vi "Kinesis - KPZ101 - Waveform LUT.vi"() -> ()   [LabVIEW 2012]
uses:
  U:/Kinesis LabVIEW Website Examples/Thorlabs.MotionControl.Controls.dll
  Thorlabs.MotionControl.Controls.dll
  U:/Kinesis LabVIEW Website Examples/Thorlabs.MotionControl.GenericPiezoCLI.dll
  Thorlabs.MotionControl.GenericPiezoCLI.dll
  <vilib>/measure/NI_MABase.lvlib
  U:/Kinesis LabVIEW Website Examples/Thorlabs.MotionControl.KCube.PiezoCLI.dll
  Thorlabs.MotionControl.KCube.PiezoCLI.dll
panel:
  in  "?":bool
  in  "?":bool
  in  "Milliseconds to Stop":u32=10000
  out "Sine Wave Array":dbl[](array[numeric])
  in  "Peak Voltage":dbl=5.0
  in  "SerialNumber":string
  in  "NumberOfCycles":u32
  in  "Mode":i16(ring)=1 items=["Continuous"=1, "Fixed"=2, "OutputTrigEnable"=4, "InputTrigEnable"=8, "OutputTrigSenseHigh"=16, "InputTrigSenseHigh"=32, "OutputGated"=64, "OutputTrigRepeat"=128]
  in  "LUTValDelay":u32=10
  in  "PostCycleDelay":u32=5
  in  "PreCycleDelay":u32=5
  in  "KCubePiezoControl":refnum<k24>(container)
  # "Notes:"
  # "- Ensure that the appropriate .DLLs are copied into your Project Folder. Check that the correct bit type are used depending on your version of LabVIEW\ni.e. 32-bit or 64-bit.\n\n\n\n\n\n\n\n\n\n\n\n\n\n\n- Open the example VI through the LabVIEW Project Explorer to correctly load the User Interface from Thorlabs.MotionControl.Controls.dll."
  # "Thorlabs Hardware: KPZ101 - K-Cube Piezo Controller\nhttps://www.thorlabs.com/newgrouppage9.cfm?objectgroup_id=2421&pn=KPZ101\n\nDescription: This VI will enable you to make use of the LUTWave Functionality available to Piezo actuated device. \nTaking advantage of the built-in Sine Waveform.vi of LabVIEW, we produce an array of sine wave component values, \nscaled by the Peak Voltage parameter below to produce our waveform. The sine wave period is represented by 50 indexed values in the array.\nUsers are then prompted to select parameters of the LUTWaveParams() struct below the UI before initiating the waveform by clicking 'GO'.\nThe below settings will output the waveform continuously until a 10 second timer has elapsed.\n\nInstructions: \n1) Connect your KPZ101 device to your PC & ensure it is powered on & the Output Enabled. \nFor full device setup, the device product manual can be found on our website here. - https://www.thorlabs.com/thorproduct.cfm?partnumber=KPZ101 \n2) Enter the device serial number below.\n3) Click 'Run' in the LabVIEW Toolbar.\n4) Assign a timer for 'Milliseconds to Stop' as a timeout for when the Waveform should stop.\n5) Assign Parameters to the Waveform & then Click 'GO' - this will print the sine wave array to the front panel & then start the waveform output.\n6) Click 'STOP' to end the program."
  # "Example Image of .NET Controller - VI opened via Project Explorer/ not opened via Project Explorer"
  # "VI Not Opened via Project Explorer"
  # "VI Opened via Project Explorer"
  # "Time before next cycle starts"
  # "Number of times to repeat cycles"
  # "- To explore the range of methods available, please visit the .NET API, included with your Kinesis software.\n\n- For tips on building your own VIs with Thorlabs Motion Control Hardware, please see our LabVIEW Guide here.\nhttps://www.thorlabs.com/newgrouppage9.cfm?objectgroup_id=10285"
  # "Time after cycle finishes"
  # "Time between output updates"
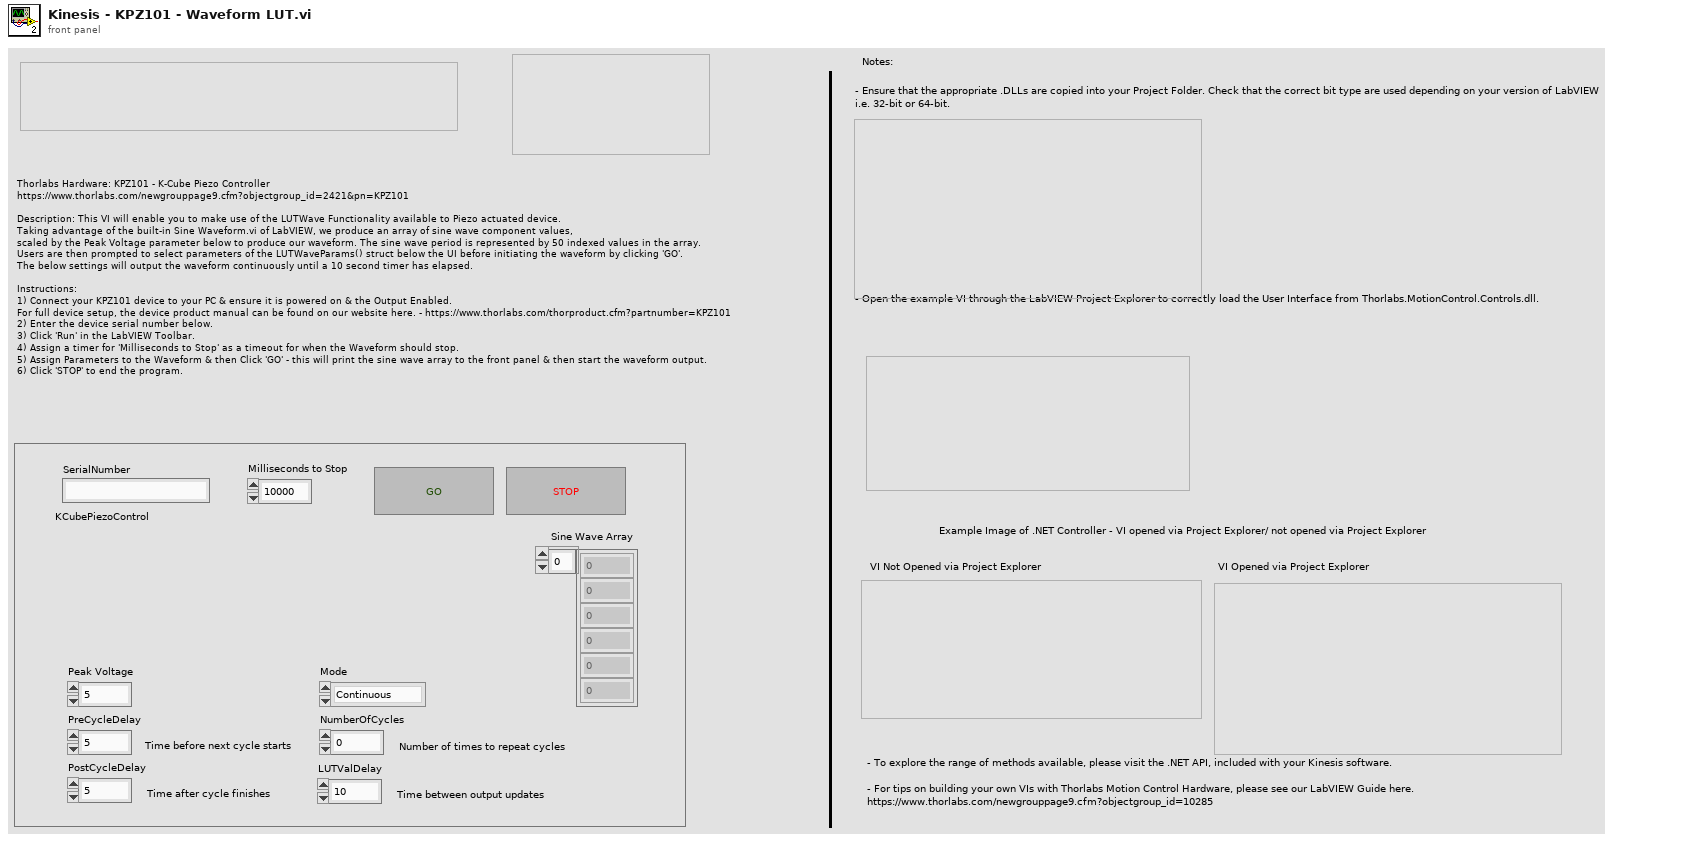
[diagram p1: front panel]
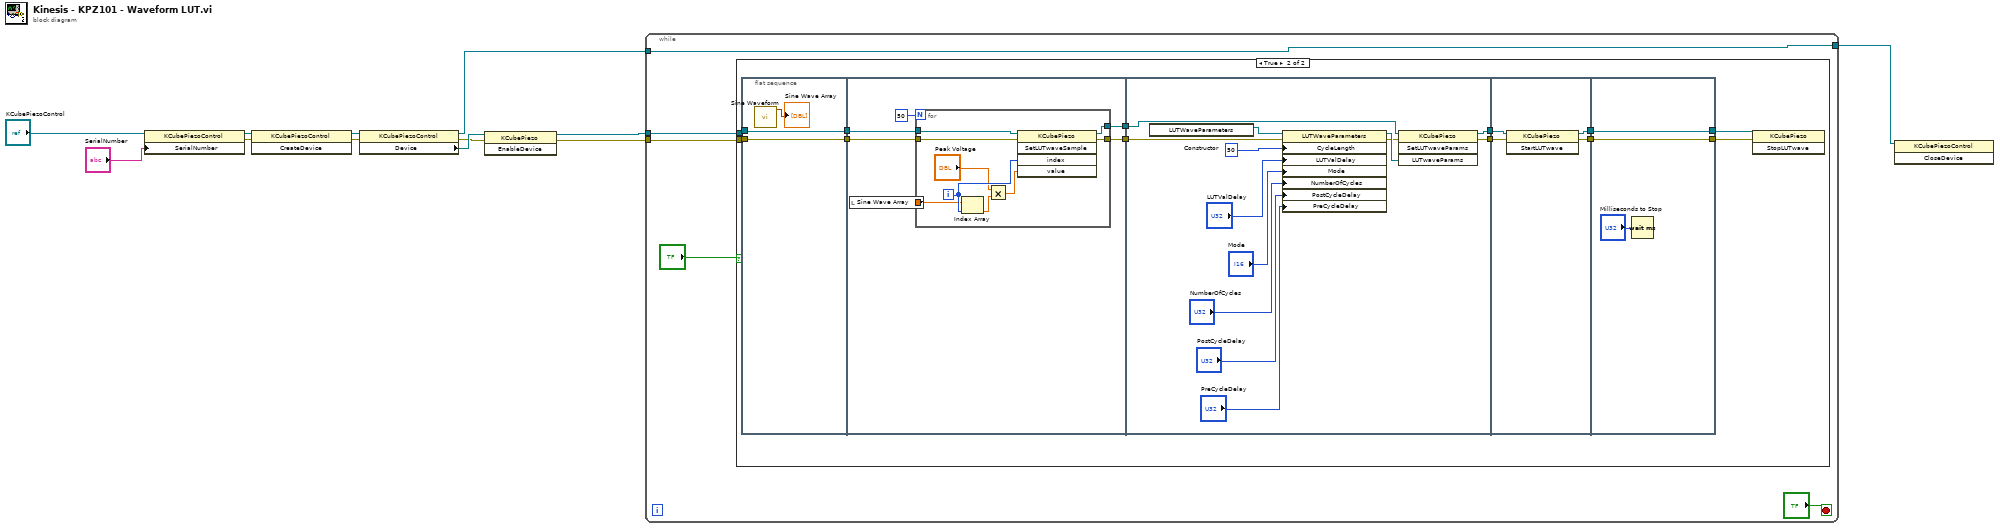
[diagram p0: block diagram]
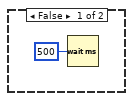
[diagram p2: hidden frame]
diagram:
  n1 = property class="KCubePiezoControl"(reference="KCubePiezoControl", "SerialNumber"="SerialNumber") -> (reference out=w11:refnum<k24>, error out=w7:errorcluster)  [unwired: 1 in]
  n2 = invoke class="KCubePiezoControl" method="CreateDevice"(reference=w11, error in=w7) -> (reference out=w10:refnum<k24>, error out=w6:errorcluster)  [unwired: 1 in, 1 out]
  n3 = property class="KCubePiezoControl"(reference=w10, error in=w6) -> (reference out=w4:refnum<k24>, error out=w5:errorcluster, "Device"=w9:refnum<k24>)
  n4 = invoke class="KCubePiezo" method="EnableDevice"(reference=w9, error in=w5) -> (reference out=w2:refnum<k24>, error out=w1:errorcluster)  [unwired: 1 in, 1 out]
  n5 = while {
    tunnel: w4 -> [w16]
    tunnel: [w16] -> w3
    tunnel: w2 -> [w15]
    tunnel: w1 -> [w14]
    stop <- "?" stop-if-true
    n6 = case shown="True" "?" {
      tunnel: w15 -> [_ w20]
      tunnel: w14 -> [_ w19]
      frame False {
        n7 = Wait (ms)(milliseconds to wait=u32 500) -> ()  [unwired: 1 out]
      }
      frame True {
        n8 = flat-sequence {
          tunnel: w20 -> [w33]
          tunnel: [w33] -> w30
          tunnel: [w31] -> w29
          tunnel: w19 -> [w31]
          tunnel: [w36] -> w28
          tunnel: w30 -> [w37]
          tunnel: w29 -> [w35]
          tunnel: [w34] -> w27
          tunnel: w28 -> [w55]
          tunnel: [w61] -> w26
          tunnel: w27 -> [w52]
          tunnel: [w50] -> w25
          tunnel: w26 -> [w65]
          tunnel: w25 -> [w63]
          tunnel: [w64] -> w24
          tunnel: [w62] -> w23
          tunnel: [w67] -> w21
          tunnel: [w68] -> w22
          tunnel: w24 -> [w68]
          tunnel: w23 -> [w67]
          frame #0 {
            n9 = call <vilib>:"Sine Waveform.vi"() -> ("signal out"=→"Sine Wave Array":waveform(dbl))  [unwired: 10 in, 1 out]
          }
          frame #1 {
            n10 = local read "Sine Wave Array"() -> (w38:dbl[])
            n11 = for {
              N: 50 -> [_]
              tunnel: w37 -> [w45]
              tunnel: [w44] -> w36
              tunnel: w35 -> [w42]
              tunnel: [w41] -> w34
              tunnel: w38 -> [w40]
              i -> [w48]
              n12 = Index Array(array=w40, index=w48) -> (element=w47:dbl)
              n13 = Multiply(x="Peak Voltage", y=w47) -> (x*y=w43:dbl)
              n14 = invoke class="KCubePiezo" method="SetLUTwaveSample"(reference=w45, error in=w42, "index"=w48, "value"=w43) -> (reference out=w44:refnum<k24>, error out=w41:errorcluster)  [unwired: 1 in, 3 out]
            }
          }
          frame #2 {
            n15 = constructor class="LUTWaveParameters"() -> (reference out=w53:refnum<k24>)  [unwired: 3 in, 2 out]
            n16 = property class="LUTWaveParameters"(reference=w53, error in=w52, "CycleLength"=i16 50, "LUTValDelay"="LUTValDelay", "Mode"="Mode", "NumberOfCycles"="NumberOfCycles", "PostCycleDelay"="PostCycleDelay", "PreCycleDelay"="PreCycleDelay") -> (reference out=w54:refnum<k24>, error out=w51:errorcluster)
            n17 = invoke class="KCubePiezo" method="SetLUTwaveParams"(reference=w55, error in=w51, "LUTwaveParams"=w54) -> (reference out=w61:refnum<k24>, error out=w50:errorcluster)  [unwired: 1 in, 2 out]
          }
          frame #3 {
            n18 = invoke class="KCubePiezo" method="StartLUTwave"(reference=w65, error in=w63) -> (reference out=w64:refnum<k24>, error out=w62:errorcluster)  [unwired: 1 in, 1 out]
          }
          frame #4 {
            n19 = Wait (ms)(milliseconds to wait="Milliseconds to Stop") -> ()  [unwired: 1 out]
          }
        }
        n20 = invoke class="KCubePiezo" method="StopLUTwave"(reference=w22, error in=w21) -> ()  [unwired: 1 in, 3 out]
      }
    }
  }
  n21 = invoke class="KCubePiezoControl" method="CloseDevice"(reference=w3) -> ()  [unwired: 2 in, 3 out]
